vi "Do Action.vi"(8 "error in (no error)":errorcluster, 9 "Display Queue":refnum<queue>, 10 "tlc_User Event Reference.ctl":T1, 11 "Load in":refnum<class "Load.lvclass">) -> (0 "error out":errorcluster)   [LabVIEW 2010, in "Load.lvclass"]
doc: "This instance of Do Action.vi is used to perform the functionality that was previously contained in the Load case of the consumer loop. The file path obtained in the producer loop is used to specify the file that will be loaded to the Cue List on the UI of TLC Main.vi."
uses:
  Load.lvclass
  Controls/tlc_User Interface Command.ctl
  Controls/tlc_User Interface Data Type.ctl
  Controls/tlc_User Event Reference.ctl
  Load.lvclass/Load.ctl
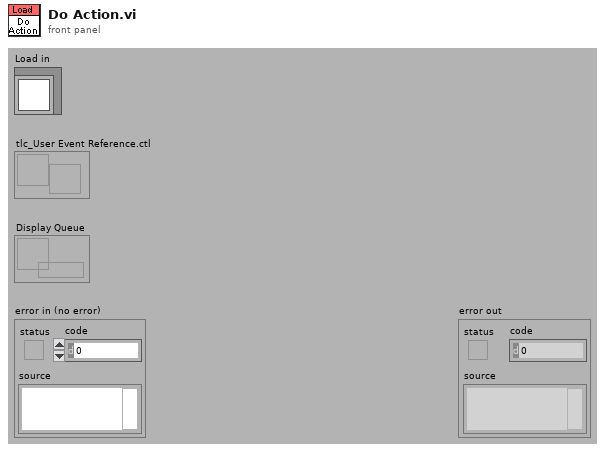
[diagram p1: front panel]
types:
  T1 = typedef "tlc_User Event Reference.ctl" = refnum<user-event>
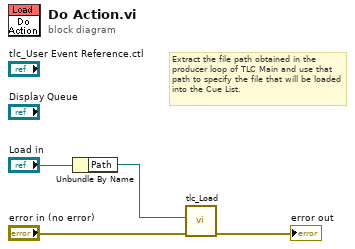
[diagram p0: block diagram]
diagram:
  # "Extract the file path obtained in the producer loop of TLC Main and use that path to specify the file that will be loaded into the Cue List."
  n1 = Unbundle By Name "Unbundle By Name"("Load in") -> ("Path"=w1:path)
  n2 = call "tlc_Load.vi"("error in (no error)"="error in (no error)", "Path"=w1) -> ("error out"=→"error out":errorcluster)  [unwired: 9 in]
